vi "Make_RDDF(UTM).vi"() -> ()   [LabVIEW 2024]
uses:
  <vilib>/Utility/file.llb/Read Delimited Spreadsheet (DBL).vi
  <vilib>/Utility/file.llb/Write Delimited Spreadsheet (DBL).vi
  <vilib>/Instr/_visa.llb/VISA Configure Serial Port (Instr).vi
panel:
  out "Display_Long":dbl
  out "Display_Lat":dbl
  in  "COM4":refnum<visa-resource-name>="COM7" caption="F9P_USB"
  out "SOG(kph)":dbl format="%#_12g"
  in  "입력속도":dbl=5.0 format="%#_13g"
  out "UTM X(N) INS":dbl format="%#_13g"
  out "UTM Y(E) INS":dbl format="%#_13g"
  out "True_Heading":dbl format="%#_15g"
  in  "Stop":bool
  in  "file path (dialog if empty)":path caption="파일 경로(비었을 경우 대화 상자 창)"
  in  "dist.":dbl=0.2
  in  "Evt":bool
  out "XY 그래프":cluster{dbl[], dbl[]}[](graph)
  in  "File_Name(User):":string
  out "File_Name(Save):":string
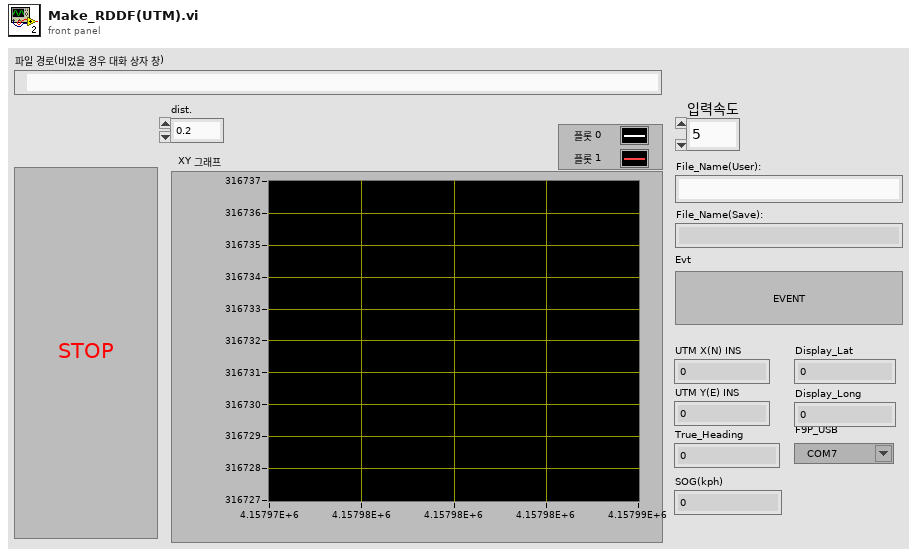
[diagram p1: front panel]
types:
  T1 = cluster{"oldest read timestamp":dbl, "latitude (deg)":dbl, "longitude (deg)":dbl, "ground speed (kph)":dbl, "true track angle (deg)":dbl, "altitude above mean sea level (m)":dbl}
  T2 = enum16{"open", "replace", "create", "open or create", "replace or create", "replace or create with confirmation"}
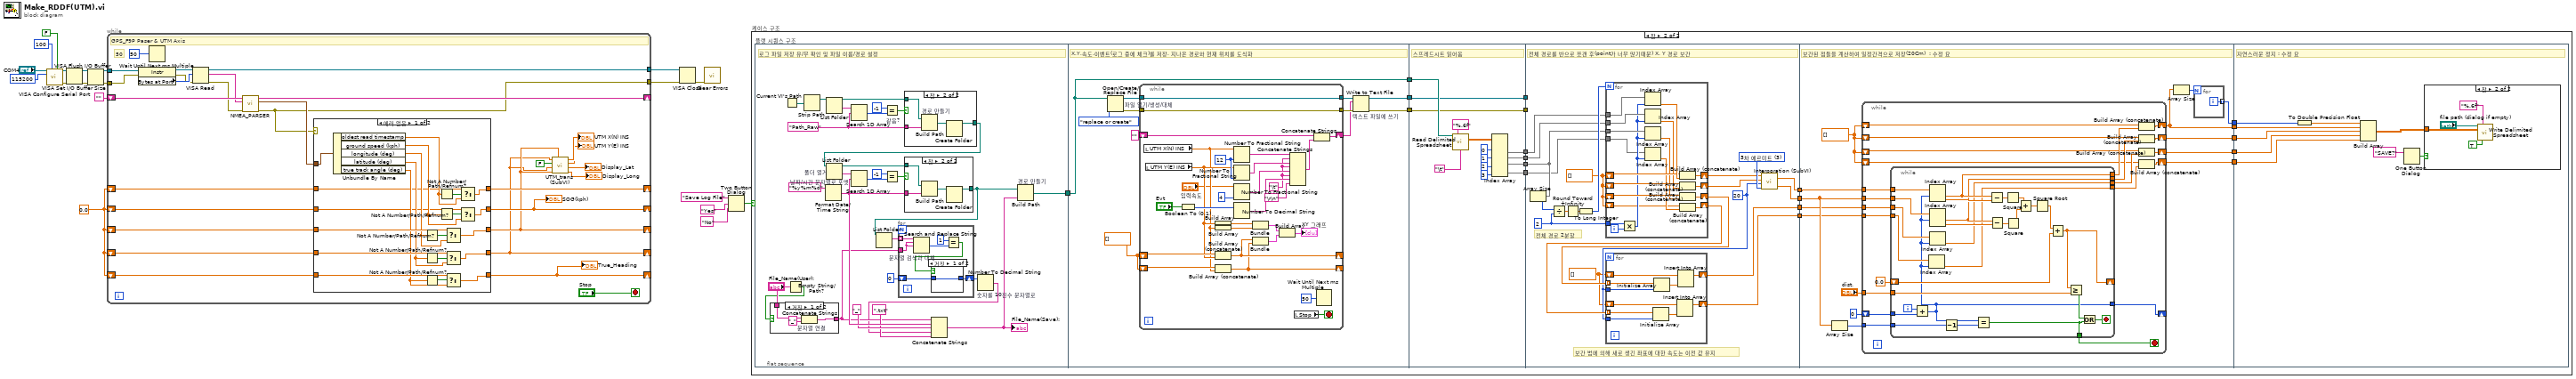
[diagram p0: block diagram]
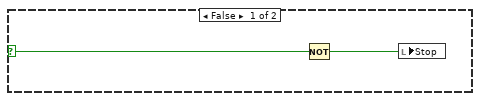
[diagram p3: hidden frame]
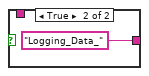
[diagram p4: hidden frame]
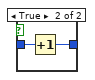
[diagram p5: hidden frame]
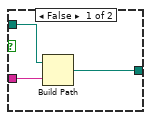
[diagram p6: hidden frame]
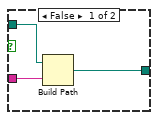
[diagram p7: hidden frame]
diagram:
  w2 = 0.0 ("x")
  n1 = call-poly "VISA Configure Serial Port"("VISA resource name"="COM4", "timeout (10sec)"=u32 100, "Enable Termination\nChar (T)"=FALSE ("Enable Termination\nChar (T)"), "baud rate (9600)"=u32 115200) -> ("VISA resource name out"=w13:refnum<visa-resource-name>, "error out"=w12:errorcluster)  [unwired: 10 in]
  n2 = VISA Set I/O Buffer Size(VISA resource name=w13, error in (no error)=w12) -> (VISA resource name out=w8:refnum<visa-resource-name>, error out=w7:errorcluster)  [unwired: 2 in]
  n3 = VISA Flush I/O Buffer(VISA resource name=w8, error in (no error)=w7) -> (VISA resource name out=w6:refnum<visa-resource-name>, error out=w5:errorcluster)  [unwired: 1 in]
  n4 = while {
    tunnel: w6 -> [w46]
    tunnel: w5 -> [w44]
    tunnel: [w48] -> w11
    tunnel: [w36] -> w9
    shift-right: [w37] -> _
    shift-left: "" -> [w41]
    shift-right: [w28] -> _
    shift-left: w2 -> [w35]
    shift-right: [w21] -> _
    shift-left: w2 -> [w34]
    shift-right: [w20] -> _
    shift-left: w2 -> [w33]
    shift-right: [w25] -> _
    shift-left: w2 -> [w32]
    shift-right: [w29] -> _
    shift-left: w2 -> [w31]
    stop <- "Stop" stop-if-true
    # "50"
    # "GPS_F9P Paser & UTM Axis"
    n5 = property class="Instr"(reference=w46, error in=w44) -> (reference out=w45:refnum<visa-resource-name>, error out=w43:errorcluster, "Bytes at Port"=w47:u32)
    n6 = Wait Until Next ms Multiple(millisecond multiple=u32 50) -> ()  [unwired: 1 out]
    n7 = VISA Read(VISA resource name=w45, byte count=w47, error in (no error)=w43) -> (VISA resource name out=w48:refnum<visa-resource-name>, read buffer=w40:string, error out=w38:errorcluster)  [unwired: 1 out]
    n8 = call "NMEA_PARSER.vi"("previous partial sentence"=w41, "sensor data"=w40, "error in (no error)"=w38) -> ("remaining partial sentence"=w37:string, "GPS data"=w39:T1, "error out"=w36:errorcluster)  [unwired: 5 in]
    n9 = case shown="에러 없음" w36 {
      tunnel: w39 -> [w69 _]
      tunnel: w34 -> [w65 w74]
      tunnel: w33 -> [w64 w73]
      tunnel: w32 -> [w63 w72]
      tunnel: [w59 w74] -> w21
      tunnel: [w58 w73] -> w20
      tunnel: [w57 w72] -> w25
      tunnel: w35 -> [w54 w71]
      tunnel: [w53 w71] -> w28
      tunnel: w31 -> [w50 w70]
      tunnel: [w49 w70] -> w29
      frame No Error {
        n10 = Unbundle By Name(w69) -> ("oldest read timestamp"=w51:dbl, "ground speed (kph)"=w55:dbl, "longitude (deg)"=w62:dbl, "latitude (deg)"=w61:dbl, "true track angle (deg)"=w60:dbl)
        n11 = Not A Number/Path/Refnum?(number/path/refnum=w62) -> (NaN/Path/Refnum?=w68:bool)
        n12 = Not A Number/Path/Refnum?(number/path/refnum=w61) -> (NaN/Path/Refnum?=w67:bool)
        n13 = Not A Number/Path/Refnum?(number/path/refnum=w60) -> (NaN/Path/Refnum?=w66:bool)
        n14 = Not A Number/Path/Refnum?(number/path/refnum=w51) -> (NaN/Path/Refnum?=w52:bool)
        n15 = Not A Number/Path/Refnum?(number/path/refnum=w55) -> (NaN/Path/Refnum?=w56:bool)
        n16 = Select(t=w65, s=w68, f=w62) -> (s? t:f=w59:dbl)
        n17 = Select(t=w64, s=w67, f=w61) -> (s? t:f=w58:dbl)
        n18 = Select(t=w63, s=w66, f=w60) -> (s? t:f=w57:dbl)
        n19 = Select(t=w50, s=w52, f=w51) -> (s? t:f=w49:dbl)
        n20 = Select(t=w54, s=w56, f=w55) -> (s? t:f=w53:dbl)
      }
      frame Error {
        # "Invalid data points."
      }
    }
    "SOG(kph)" <- w28
    "True_Heading" <- w25
    n21 = call "UTM_trans (SubVI).vi"("Long_Deg"=w21, "long"=w21, "lat"=w20, "East?West?"=FALSE, "Lat_Deg"=w20) -> ("Display_Long"=→"Display_Long":dbl, "Display_Lat"=→"Display_Lat":dbl, "UTM_Y(Northing)"=→"UTM Y(E) INS":dbl, "UTM_X(Easting)"=→"UTM X(N) INS":dbl)
  }
  n22 = VISA Close(VISA resource name=w11, error in (no error)=w9) -> (error out=w10:errorcluster)
  n23 = call <vilib>:"Clear Errors.vi"("error in (no error)"=w10) -> ()  [unwired: 5 in, 2 out]
  n24 = Two Button Dialog(message="Save Log File" ("메시지"), 1:"No" ("거짓 버튼 이름(\"취소\")"), 2:"Yes" ("참 버튼 이름(\"확인\")")) -> (T button?=w16:bool)
  n25 = case "케이스 구조" shown="참" w16 {
    selector: w16 -> [w76 _]
    frame False {
      n26 = Not(x=w76) -> (.not. x?=w75:bool)
      n27 = local write "Stop"(w75) -> ()
    }
    frame True {
      n28 = flat-sequence "플랫 시퀀스 구조" {
        tunnel: [w123] -> w95
        tunnel: w95 -> [w155]
        tunnel: [w155] -> w94
        tunnel: [w154] -> w93
        tunnel: [w153] -> w92
        tunnel: w94 -> [w205]
        tunnel: w93 -> [w201]
        tunnel: w92 -> [w202]
        tunnel: [w202] -> w90
        tunnel: [w201] -> w89
        tunnel: [w194] -> w88
        tunnel: [w195] -> w87
        tunnel: [w199] -> w86
        tunnel: [w192] -> w79
        tunnel: [w217] -> w91
        tunnel: w90 -> [_]
        tunnel: w89 -> [_]
        tunnel: w88 -> [w219]
        tunnel: w87 -> [w220]
        tunnel: w86 -> [w221]
        tunnel: [w213] -> w85
        tunnel: [w212] -> w84
        tunnel: w79 -> [w211]
        tunnel: [w206] -> w78
        tunnel: w91 -> [w263]
        tunnel: w85 -> [w265]
        tunnel: w84 -> [w264]
        tunnel: [w262] -> w83
        tunnel: [w261] -> w82
        tunnel: [w260] -> w81
        tunnel: [w259] -> w80
        tunnel: w78 -> [w258]
        tunnel: [w256] -> w77
        tunnel: w83 -> [w327]
        tunnel: w82 -> [w322]
        tunnel: w81 -> [w323]
        tunnel: w80 -> [w324]
        tunnel: w77 -> [w321]
        frame #0 {
          w118 = "Path_Raw" ("원소")
          # "로그 파일 저장 유/무 확인 및 파일 이름/경로 설정"
          n29 = Current VI's Path ("현재 VI의 경로")() -> (path=w122:path)
          n30 = Empty String/Path? ("빈 문자열/경로?")(string/path="File_Name(User):") -> (empty?=w98:bool)
          n31 = case shown="거짓" w98 {
            tunnel: [w125 "Logging_Data_"] -> w102
            tunnel: "File_Name(User):" -> [w124 _]
            frame False {
              n32 = Concatenate Strings "문자열 연결"(w124, "_" ("문자열")) -> (w125:string)
            }
            frame True {
            }
          }
          n33 = Strip Path ("경로 분리")(path=w122) -> (stripped path=w121:path)  [unwired: 1 out]
          n34 = Format Date/Time String "날짜/시간 문자열로 포맷"(time format string (%c)="%y%m%d" ("시간 포맷 문자열 (%c)")) -> (date/time string=w105:string)  [unwired: 2 in]
          n35 = List Folder ("폴더 열거")(path=w121) -> (path out=w120:path, folder names=w117:string[])  [unwired: 3 in, 2 out]
          n36 = Search 1D Array ("1D 배열 검색")(1D array=w117, element=w118) -> (index of element=w116:i32)  [unwired: 1 in]
          n37 = Equal? "같음?"(x=-1 ("y"), y=w116) -> (x = y?=w119:bool)
          n38 = case shown="참" w119 {
            tunnel: w120 -> [w145 w150]
            tunnel: w118 -> [w146 w149]
            tunnel: [w147 w148] -> w108
            frame False {
              n39 = Build Path ("경로 만들기")(base path=w145, name or relative path=w146) -> (appended path=w147:path)
            }
            frame True {
              n40 = Build Path "경로 만들기"(base path=w150, name or relative path=w149) -> (appended path=w151:path)
              n41 = Create Folder ("폴더 생성")(path (use dialog)=w151) -> (created path=w148:path)  [unwired: 2 in, 2 out]
            }
          }
          n42 = List Folder "폴더 열거"(path=w108) -> (path out=w109:path, folder names=w111:string[])  [unwired: 3 in, 2 out]
          n43 = Search 1D Array(1D array=w111, element=w105) -> (index of element=w112:i32)  [unwired: 1 in]
          n44 = Equal?(x=-1 ("y"), y=w112) -> (x = y?=w110:bool)
          n45 = case shown="참" w110 {
            tunnel: w109 -> [w138 w143]
            tunnel: w105 -> [w139 w142]
            tunnel: [w140 w141] -> w97
            frame False {
              n46 = Build Path(base path=w138, name or relative path=w139) -> (appended path=w140:path)
            }
            frame True {
              n47 = Build Path(base path=w143, name or relative path=w142) -> (appended path=w144:path)
              n48 = Create Folder(path (use dialog)=w144) -> (created path=w141:path)  [unwired: 2 in, 2 out]
            }
          }
          n49 = List Folder ("폴더 열거")(path=w97) -> (filenames=w107:string[])  [unwired: 3 in, 3 out]
          n50 = for {
            tunnel: w107 -> [w134] mode=indexing
            shift-right: [w129] -> w101
            shift-left: 0 -> [w130]
            tunnel: w102 -> [w128]
            n51 = Search and Replace String "문자열 검색과 대체"(input string=w134, search string=w128, replace string=w128) -> (number of replacements=w132:i32)  [unwired: 5 in, 3 out]
            n52 = Equal?(x=1, y=w132) -> (x = y?=w131:bool)
            n53 = case shown="거짓" w131 {
              tunnel: w130 -> [w135 w137]
              tunnel: [w135 w136] -> w129
              frame False {
              }
              frame True {
                n54 = Increment(x=w137) -> (x+1=w136:i32)
              }
            }
          }
          n55 = Number To Decimal String "숫자를 10진수 문자열로"(number=w101) -> (decimal integer string=w100:string)  [unwired: 1 in]
          n56 = Concatenate Strings(w102, w105, "_" ("문자열"), w100, ".txt" ("문자열")) -> (w96:string)
          "File_Name(Save):" <- w96
          n57 = Build Path "경로 만들기"(base path=w97, name or relative path=w96) -> (appended path=w123:path)
        }
        frame #1 {
          w152 = dbl[] []
          # "X,Y,속도,이벤트(로그 중에 체크)를 저장, 지나온 경로와 현재 위치를 도식화"
          n58 = Open/Create/Replace File "파일 열기/생성/대체"(file path (use dialog)=w155, operation (0:open)=T2."replace or create" ("동작(0:open)")) -> (refnum out=w160:refnum<file>, error out=w161:errorcluster)  [unwired: 4 in, 1 out]
          n59 = while {
            tunnel: w161 -> [w186]
            tunnel: w160 -> [w187]
            tunnel: [w187] -> w158
            tunnel: [w186] -> w159
            shift-right: [w171] -> w157
            shift-left: "" -> [w173]
            shift-right: [w167] -> _
            shift-left: w152 -> [w178]
            shift-right: [w166] -> _
            shift-left: w152 -> [w177]
            stop <- w185 stop-if-true
            w180 = "\t"
            w191 = i16 12 ("정밀도(6)")
            n60 = local read "UTM X(N) INS"() -> (w164:dbl)
            n61 = local read "UTM Y(E) INS"() -> (w165:dbl)
            n62 = Boolean To (0,1)(Boolean="Evt") -> (0, 1=w188:i16)
            n63 = Build Array(w165) -> (w176:dbl[])
            n64 = Build Array(w164) -> (w175:dbl[])
            n65 = Build Array (concatenate)(w178, w165) -> (w167:dbl[])
            n66 = Build Array (concatenate)(w177, w164) -> (w166:dbl[])
            n67 = Number To Fractional String(number=w164, precision (6)=w191) -> (F-format string=w184:string)  [unwired: 2 in]
            n68 = Number To Fractional String(number=w165, precision (6)=w191) -> (F-format string=w183:string)  [unwired: 2 in]
            n69 = Number To Fractional String(number="입력속도", precision (6)=i16 4 ("정밀도(6)")) -> (F-format string=w182:string)  [unwired: 2 in]
            n70 = Number To Decimal String(number=w188) -> (decimal integer string=w181:string)  [unwired: 1 in]
            n71 = Bundle(w176, w175) -> (w168:cluster{dbl[], dbl[]})  [unwired: 1 in]
            n72 = Bundle(w167, w166) -> (w169:cluster{dbl[], dbl[]})  [unwired: 1 in]
            n73 = Build Array(w168, w169) -> (→"XY 그래프":cluster{dbl[], dbl[]}[])
            n74 = Concatenate Strings(w184, w180, w183, w180, w182, w180, w181, "\r\n") -> (w172:string)
            n75 = local read "Stop"() -> (w185:bool)
            n76 = Concatenate Strings(w173, w172) -> (w171:string)
            n77 = Wait Until Next ms Multiple(millisecond multiple=u32 50 ("ms 배수")) -> ()  [unwired: 1 out]
          }
          n78 = Write to Text File "텍스트 파일에 쓰기"(file (use dialog)=w158, text=w157, error in=w159) -> (refnum out=w153:refnum<file>, error out=w154:errorcluster)  [unwired: 1 in, 1 out]
        }
        frame #2 {
          # "스프레드시트 읽어옴"
          n79 = call-poly <vilib>:"Read Delimited Spreadsheet.vi"("file path (dialog if empty)"=w205, "format (%.3f)"="%.6f", "delimiter (\\t)"="\t") -> ("all rows"=w200:dbl[][])  [unwired: 7 in, 5 out]
          n80 = Index Array(array=w200, index (col) #1=0 ("비활성화된 인덱스 (열)"), index (col) #2=1 ("인덱스 (열)"), index (col) #3=2 ("인덱스 (열)"), index (col) #4=3 ("인덱스 (열)")) -> (element #1=w199:dbl[], element #2=w195:dbl[], element #3=w194:dbl[], element #4=w192:dbl[])  [unwired: 4 in]
        }
        frame #3 {
          w216 = 3 items=["최근접", "선형", "스플라인", "3차 에르미트", "라그랑지"] ("method")
          w207 = dbl[] []
          w208 = 20 ("Interpolation factor (n)")
          w210 = dbl[] []
          w222 = 2
          # "보간 법에 의해 새로 생긴 좌표에 대한 속도는 이전 값 유지"
          # "전체 경로 2분할"
          # "전체 경로를 반으로 쪼갠 후(point가 너무 많기때문) X, Y 경로 보간"
          n81 = Array Size(array=w219) -> (size(s)=w226:i32)
          n82 = Divide(x=w226, y=w222) -> (x/y=w225:dbl)
          n83 = Round Toward +Infinity(x=w225) -> (ceil(x): smallest int >= x=w224:dbl)
          n84 = To Long Integer(number=w224) -> (32bit integer=w223:i32)
          n85 = for {
            N: w223 -> [_]
            tunnel: w222 -> [w254]
            tunnel: w221 -> [w253]
            tunnel: w220 -> [w252]
            tunnel: w219 -> [w251]
            shift-right: [w248] -> w215
            shift-left: w210 -> [w249]
            shift-right: [w247] -> w214
            shift-left: w210 -> [w246]
            shift-right: [w240] -> w218
            shift-left: w210 -> [w245]
            tunnel: w211 -> [w241]
            shift-right: [w237] -> w209
            shift-left: w210 -> [w238]
            i -> [w255]
            n86 = Multiply(x=w254, y=w255) -> (x*y=w242:i32)
            n87 = Index Array(array=w253, index=w242) -> (element=w250:dbl)
            n88 = Index Array(array=w252, index=w242) -> (element=w244:dbl)
            n89 = Index Array(array=w251, index=w242) -> (element=w243:dbl)
            n90 = Index Array(array=w241, index=w242) -> (element=w239:dbl)
            n91 = Build Array (concatenate)(w249, w250) -> (w248:dbl[])
            n92 = Build Array (concatenate)(w246, w244) -> (w247:dbl[])
            n93 = Build Array (concatenate)(w245, w243) -> (w240:dbl[])
            n94 = Build Array (concatenate)(w238, w239) -> (w237:dbl[])
          }
          n95 = for {
            tunnel: w218 -> [w236] mode=indexing
            tunnel: w208 -> [w235]
            shift-right: [w234] -> w217
            shift-left: w207 -> [w233]
            tunnel: w209 -> [w230] mode=indexing
            tunnel: w208 -> [w229]
            shift-right: [w227] -> w206
            shift-left: w207 -> [w228]
            n96 = Initialize Array(w230, w229) -> (w232:dbl[])
            n97 = Initialize Array(w236, w235) -> (w231:dbl[])
            n98 = Insert Into Array(array=w228, new element=w232) -> (w227:dbl[])  [unwired: 1 in]
            n99 = Insert Into Array(array=w233, new element=w231) -> (w234:dbl[])  [unwired: 1 in]
          }
          n100 = call "Interporation (SubVI).vi"("method"=w216, "Sample"=w208, "Y_long"=w214, "X_lat"=w215) -> ("Y_long"=w212:dbl[], "X_lat"=w213:dbl[])
        }
        frame #4 {
          w257 = dbl[] []
          # "보간된 점들을 계산하여 일정간격으로 저장(20Cm)  : 수정 요"
          n101 = Array Size(array=w264) -> (size(s)=w267:i32)
          n102 = while {
            tunnel: "dist." -> [w289]
            tunnel: w265 -> [w292]
            tunnel: w264 -> [w291]
            tunnel: w263 -> [w283]
            shift-right: [w278] -> _
            shift-left: 0 -> [w288]
            shift-right: [w275] -> w259
            shift-left: w257 -> [w284]
            shift-right: [w277] -> w260
            shift-left: w257 -> [w285]
            shift-right: [w276] -> w261
            shift-left: w257 -> [w281]
            tunnel: w267 -> [w280]
            tunnel: w258 -> [w274]
            shift-right: [w272] -> w256
            shift-left: w257 -> [w271]
            stop <- w279 stop-if-true
            n103 = while {
              tunnel: w292 -> [w319]
              tunnel: w291 -> [w318]
              shift-right: [w308] -> _
              shift-left: 0.0 -> [w309]
              tunnel: w289 -> [w307]
              tunnel: [w293] -> w278
              tunnel: w288 -> [w305]
              tunnel: [w304] -> w287
              tunnel: [w303] -> w286
              tunnel: w283 -> [w302]
              tunnel: [w301] -> w282
              tunnel: w280 -> [w300]
              tunnel: [w297] -> w279
              tunnel: w274 -> [w294]
              tunnel: [w295] -> w273
              i -> [w306]
              stop <- w299 stop-if-true
              n104 = Add(x=w306, y=w305) -> (x+y=w293:i32)
              n105 = Index Array(array=w294, index=w293) -> (element=w295:dbl)
              n106 = Index Array(array=w319, index #1=w293) -> (element #1=w304:dbl, element #2=w317:dbl)  [unwired: 1 in]
              n107 = Index Array(array=w318, index #1=w293) -> (element #1=w303:dbl, element #2=w316:dbl)  [unwired: 1 in]
              n108 = Index Array(array=w302, index=w293) -> (element=w301:dbl)
              n109 = Decrement(x=w300) -> (x-1=w296:i32)
              n110 = Equal?(x=w293, y=w296) -> (x = y?=w297:bool)
              n111 = Subtract(x=w304, y=w317) -> (x-y=w315:dbl)
              n112 = Subtract(x=w303, y=w316) -> (x-y=w314:dbl)
              n113 = Square(x=w315) -> (x^2=w313:dbl)
              n114 = Square(x=w314) -> (x^2=w312:dbl)
              n115 = Add(x=w313, y=w312) -> (x+y=w311:dbl)
              n116 = Square Root(x=w311) -> (sqrt(x)=w310:dbl)
              n117 = Add(x=w310, y=w309) -> (x+y=w308:dbl)
              n118 = Greater Or Equal?(x=w308, y=w307) -> (x >= y?=w298:bool)
              n119 = Or(x=w298, y=w297) -> (x .or. y?=w299:bool)
            }
            n120 = Build Array (concatenate)(w284, w287) -> (w275:dbl[])
            n121 = Build Array (concatenate)(w285, w286) -> (w277:dbl[])
            n122 = Build Array (concatenate)(w281, w282) -> (w276:dbl[])
            n123 = Build Array (concatenate)(w271, w273) -> (w272:dbl[])
          }
          n124 = Array Size(array=w259) -> (size(s)=w266:i32)
          n125 = for {
            N: w266 -> [_]
            tunnel: [w270] -> w262 mode=indexing
            i -> [w270]
          }
        }
        frame #5 {
          # "자연스러운 정지 : 수정 요"
          n126 = To Double Precision Float(number=w327) -> (double precision float=w320:dbl[])
          n127 = Build Array(w320, w324, w323, w322, w321) -> (w328:dbl[][])
          n128 = One Button Dialog(message="SAVE?") -> (true=w326:bool)  [unwired: 1 in]
          n129 = case shown="참" w326 {
            tunnel: w328 -> [_ w332]
            frame False {
            }
            frame True {
              n130 = call-poly <vilib>:"Write Delimited Spreadsheet.vi"("file path (dialog if empty)"="file path (dialog if empty)", "format (%.3f)"="%.6f", "2D data"=w332, "transpose? (no:F)"=TRUE) -> ()  [unwired: 10 in, 2 out]
            }
          }
        }
      }
    }
  }
